vi "Identify running VIs.vi"() -> (3 "Running VI":string[](array[string]))   [LabVIEW 2021]
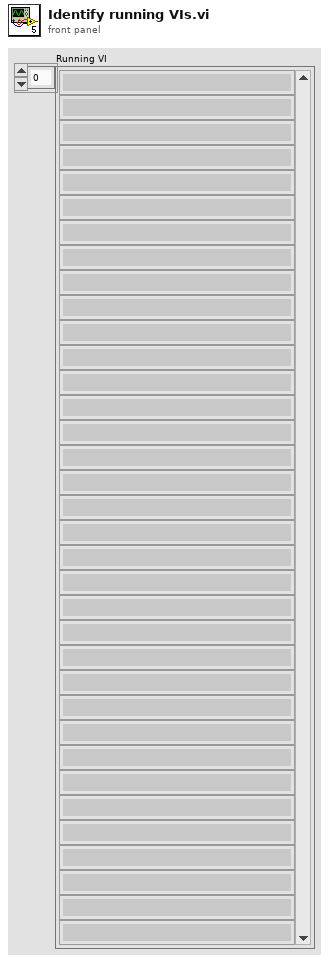
[diagram p1: front panel]
types:
  T1 = enum32{"Bad", "Idle", "Run top level", "Running"}
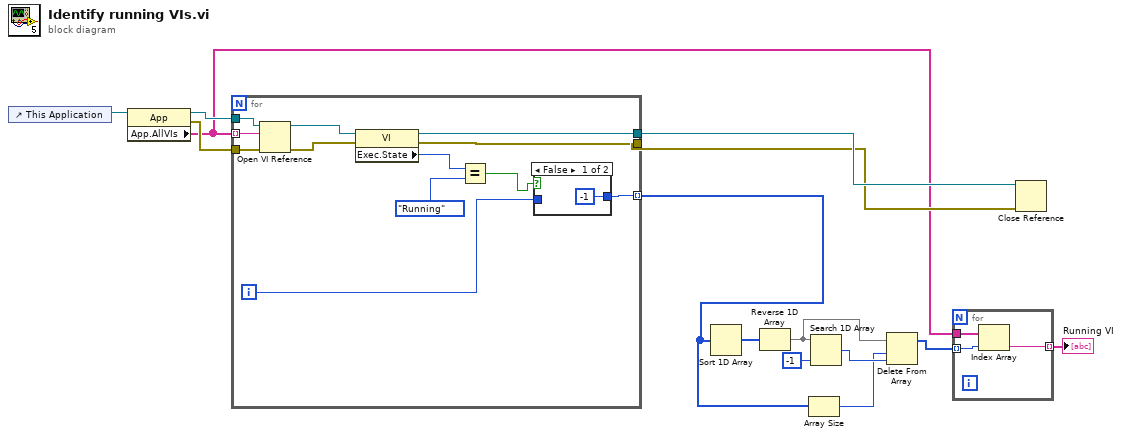
[diagram p0: block diagram]
diagram:
  n1 = control-ref of="This Application"() -> (w14:refnum<vi>)
  n2 = property class="App"(reference=w14) -> (reference out=w13:refnum<vi>, error out=w12:errorcluster, "App.AllVIs"=w1:string[])  [unwired: 1 in]
  n3 = for {
    tunnel: w1 -> [w17] mode=indexing
    tunnel: w13 -> [w26]
    tunnel: w12 -> [w25]
    tunnel: [w22] -> w11
    tunnel: [w21] -> w10
    tunnel: [w19] -> w2 mode=indexing
    i -> [w18]
    n4 = Open VI Reference(application reference (local)=w26, vi path=w17, error in (no error)=w25) -> (vi reference=w24:refnum<vi>, error out=w23:errorcluster)  [unwired: 3 in]
    n5 = property class="VI"(reference=w24, error in=w23) -> (reference out=w22:refnum<vi>, error out=w21:errorcluster, "Exec.State"=w16:T1)
    n6 = Equal?(x=w16, y=T1."Running" ("Execution:State")) -> (x = y?=w15:bool)
    n7 = case shown="False" w15 {
      tunnel: [-1 w28] -> w19
      tunnel: w18 -> [_ w28]
      frame False {
      }
      frame True {
      }
    }
  }
  n8 = Sort 1D Array(array=w2) -> (sorted array=w9:i32[])
  n9 = Reverse 1D Array(array=w9) -> (reversed array=w5:i32[])
  n10 = Array Size(array=w2) -> (size(s)=w6:i32)
  n11 = Search 1D Array(1D array=w5, element=-1) -> (index of element=w7:i32)  [unwired: 1 in]
  n12 = Delete From Array(array=w5, length=w6, index=w7) -> (array with subset deleted=w4:i32[])  [unwired: 1 out]
  n13 = for {
    tunnel: w1 -> [w31]
    tunnel: w4 -> [w30] mode=indexing
    tunnel: [w29] -> w3 mode=indexing
    n14 = Index Array(array=w31, index=w30) -> (element=w29:string)
  }
  "Running VI" <- w3
  n15 = Close Reference(reference=w11, error in (no error)=w10) -> ()  [unwired: 1 out]
